vi "BRig_comm_TCP_constants_byteRange_letters__checkRange.vi"(11 "input_byte":u8) -> (0 "output_letters_uppercase":bool, 1 "output_letters_lowercase":bool, 3 "output_letters":bool)   [LabVIEW 2014]
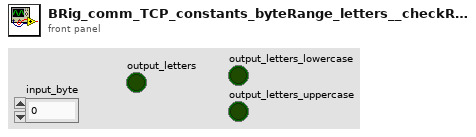
[diagram p1: front panel]
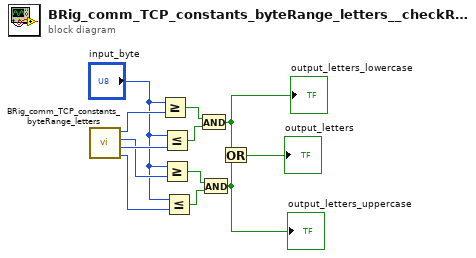
[diagram p0: block diagram]
diagram:
  n1 = call "BRig_comm_TCP_constants_byteRange_letters.vi"() -> ("output_byte_end_uppercase"=w5:u8, "output_byte_end_lowercase"=w9:u8, "output_byte_start_uppercase"=w6:u8, "output_byte_start_lowercase"=w10:u8)  [unwired: 8 in]
  n2 = Greater Or Equal?(x="input_byte", y=w10) -> (x >= y?=w12:bool)
  n3 = Less Or Equal?(x="input_byte", y=w9) -> (x <= y?=w11:bool)
  n4 = Greater Or Equal?(x="input_byte", y=w6) -> (x >= y?=w8:bool)
  n5 = Less Or Equal?(x="input_byte", y=w5) -> (x <= y?=w7:bool)
  n6 = And(x=w12, y=w11) -> (x .and. y?=w3:bool)
  "output_letters_lowercase" <- w3
  n7 = And(x=w8, y=w7) -> (x .and. y?=w2:bool)
  "output_letters_uppercase" <- w2
  n8 = Or(x=w3, y=w2) -> (x .or. y?=→"output_letters":bool)
